vi "e.gate Example - ASCII Read Value.vi"(8 "Fehler (Eingang, kein Fehler)":errorcluster, 11 "IP Address":string="10.0.10.54") -> (0 "error out":errorcluster)   [LabVIEW 2016]
doc: "<B>AMC - Analytik & Messtechnik GmbH Chemnitz</B>\n\nLabVIEW Drivers for e.gate / e.pac series from Gantner Instruments\n\nThis VI demonstrates the usage of the driver by reading an analog value from the e.gate/e.pac device."
uses:
  e.gate Protocol Type.ctl
  e.gate ASCII Read Value - Double.vi
  e.gate ASCII Write Value - Integer.vi
panel:
  out "IP Address":string="10.0.10.54"
  in  "Value":i32
  in  "Write":bool
  in  "Select channel for writing":i32
  in  "Select channel for reading":i32
  out "Value":dbl(graph)
  in  "Stop":bool
  # "EXAMPLE - Ethernet ASCII communication"
  # "Write Channel"
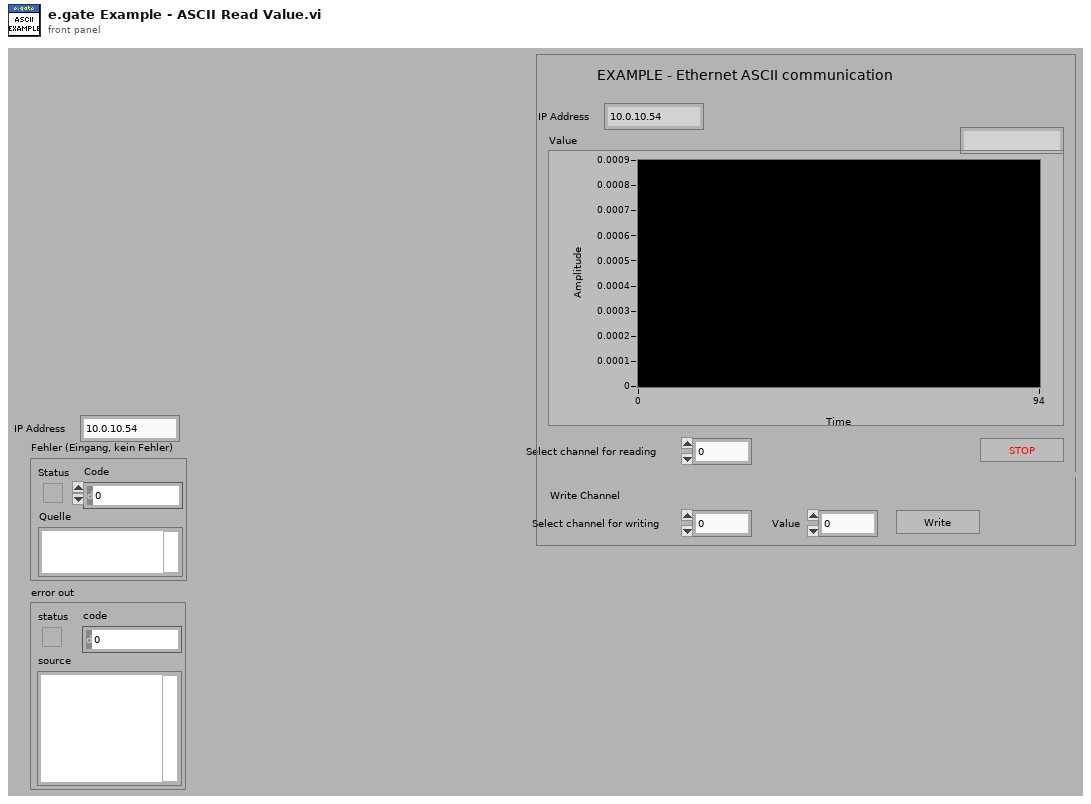
[diagram p1: front panel]
types:
  T1 = typedef "e.gate Protocol Type.ctl" = enum16{"ASCII", "HighspeedPort Online", "HighspeedPort Buffer", "eGateHighspeedPortDLL "}
  T2 = typedef "e.gate Configuration.ctl" = cluster{"connection ID":refnum<k5>, "IPAddress":string, "BufferIndex":i32, "StateMessage":string, "StateCode":i8, "HeaderSize":i32, "BufferSize":i32, "IsBigEndian":i32, "Version":i32, "ChannelCount":i32, "FrameLength":i32, "StartTime":dbl, "dActTimeToSecondFactor":dbl, "StartTimeToDayFactor":dbl, "BufferFillRate":dbl, "SampleRate":dbl, "ChannelData":T3[], "DecodeTimeFormat":string, "SummaryPath":string, "WithCheckSum":i32, "dActTimeDataType":T4, "MaxWriteCount":i32, "MaxReadCount":i32, "TempOffsetRead":i32, "TempLengthRead":i32, "Protocol":T1, "IsSupported":i32, "InputAccessList":i32[], "OutputAccessList":i32[], "DataSource":enum16{"CircleBuffer", "test.con Logger", "test.con Archive"}, "Modules":T5[], "DLL-Handle":T6}
  T3 = typedef "e.gate Channel Data.ctl" = cluster{"VariableName":string, "DataDirection":string, "DataType":string, "DataTypeIndex":T4, "Precision":i16, "FieldLengtht":i16, "ByteCount":i32, "Format":string, "Unit":string, "InputAccessOffset":i32, "OutputAccessOffset":i16, "InputAccessIndex":i16, "OutputAccessIndex":i16, "VarType":string}
  T4 = typedef "e.gate Data Type.ctl" = enum16{"NO", "BOOL", "SINT8", "USINT8", "SINT16", "USINT16", "SINT32", "USINT32", "FLOAT", "SET8", "SET16", "SET32", "DOUBLE", "SINT64", "USINT64", "SET64"}
  T5 = typedef "e.gate Module  Data.ctl" = cluster{"Type":string, "Location":string, "VariablesCount":i16, "UartIndex":i16, "Address":i16, "SystemOffset":i16}
  T6 = typedef "e.gateHSP_DLLhandle.ctl" = cluster{"clientInstance":i32, "connectionInstance":i32}
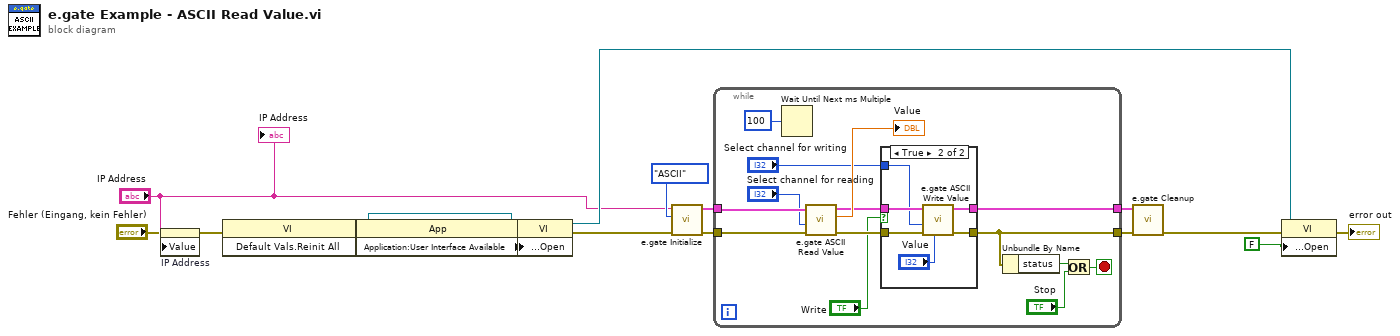
[diagram p0: block diagram]
diagram:
  n1 = property on="IP Address" class="Str"(error in="Fehler (Eingang, kein Fehler)", "Value"="IP Address") -> (error out=w1:errorcluster)  [unwired: 1 in, 1 out]
  n2 = invoke class="VI" method="Default Vals.Reinit All"(error in=w1) -> (reference out=w12:refnum<vi>, error out=w10:errorcluster)  [unwired: 2 in, 1 out]
  n3 = property class="App"(error in=w10) -> (error out=w9:errorcluster, "Application:User Interface Available"=w11:bool)  [unwired: 1 in, 1 out]
  n4 = property class="VI"(reference=w12, error in=w9, "Front Panel.Open"=w11) -> (reference out=w5:refnum<vi>, error out=w8:errorcluster)
  n5 = call "e.gate Initialize.vi"("error in (no error)"=w8, "Protocol"=e.gate_Protocol_Type."ASCII", "IP Address"="IP Address") -> ("error out"=w15:errorcluster, "e.gate Configuration"=w14:T2)  [unwired: 1 in, 6 out]
  n6 = while {
    tunnel: [w22] -> w16
    tunnel: w14 -> [w31]
    tunnel: w15 -> [w30]
    tunnel: [w20] -> w17
    stop <- w26 stop-if-true
    n7 = Wait Until Next ms Multiple(millisecond multiple=u32 100) -> ()  [unwired: 1 out]
    n8 = call-poly "e.gate ASCII Read Value.vi"("error in (no error)"=w30, "Channel"="Select channel for reading", "e.gate Configuration In"=w31) -> ("error out"=w21:errorcluster, "Value"=→"Value":dbl, "e.gate Configuration Out"=w23:T2)  [unwired: 6 out]
    n9 = case shown="True" "Write" {
      tunnel: w23 -> [w33 w39]
      tunnel: [w33 w38] -> w22
      tunnel: w21 -> [w32 w37]
      tunnel: [w32 w36] -> w20
      tunnel: "Select channel for writing" -> [_ w35]
      frame False {
      }
      frame True {
        n10 = call-poly "e.gate ASCII Write Value.vi"("Value"="Value", "error in (no error)"=w37, "Channel"=w35, "e.gate Configuration In"=w39) -> ("error out"=w36:errorcluster, "e.gate Configuration Out"=w38:T2)  [unwired: 6 out]
      }
    }
    n11 = Unbundle By Name(w20) -> ("status"=w27:bool)
    n12 = Or(x=w27, y="Stop") -> (x .or. y?=w26:bool)
  }
  n13 = call "e.gate Cleanup.vi"("error in (no error)"=w17, "e.gate Configuration"=w16) -> ("error out"=w7:errorcluster)  [unwired: 9 out]
  n14 = property class="VI"(reference=w5, error in=w7, "Front Panel.Open"=FALSE ("Frontpanel-Fenster:Öffnen")) -> (error out=→"error out":errorcluster)  [unwired: 1 out]
  "IP Address" <- "IP Address"
